vi "tcsWEP_cancelCallback_timestamp.vi"(8 "error in (no error)":errorcluster) -> (0 "error out":errorcluster, 3 "function return":i32)   [LabVIEW 2016, in "SALLV_tcsWEP.lvlib"]
doc: "int tcsWEP_shm_cancelCallback_timestampLV();"
uses:
  SALLV_tcsWEP.lvlib
  SALLV_tcsWEP.so
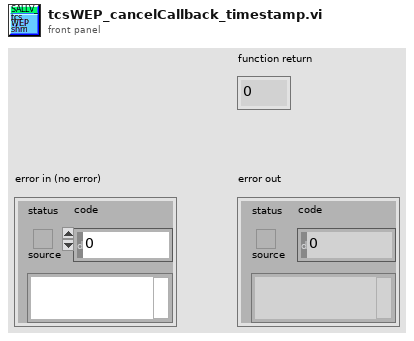
[diagram p1: front panel]
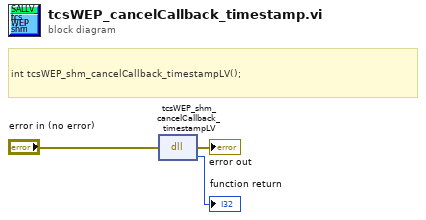
[diagram p0: block diagram]
diagram:
  # "int tcsWEP_shm_cancelCallback_timestampLV();"
  n1 = dll-call lib="home/ttsai/Documents/salAPI/SALLV_tcsWEP.*" fn="tcsWEP_shm_cancelCallback_timestampLV"(error in="error in (no error)") -> (error out=→"error out":errorcluster, →"function return":i32)  [unwired: 2 in, 1 out]
